vi "HFRR ADV v037 new software.vi"() -> ()   [LabVIEW 2025] (continued)
                      }
                      frame #18 {
                        n2411 = Wait (ms)(milliseconds to wait=u32 50) -> ()  [unwired: 1 out]
                      }
                      frame #19 {
                        n2412 = disable-structure shown="Disabled" {
                          frame Disabled {
                            n2413 = local read "EVENT LOG"() -> (w3480:string)
                            n2414 = call "Event Log.vi"("Content"="Test Parameter", "EVENT LOG"=w3480) -> ("EVENT LOG"=w3479:string)  [unwired: 8 in, 1 out]
                            n2415 = local write "EVENT LOG"(w3479) -> ()
                          }
                          frame Enabled {
                          }
                        }
                      }
                      frame #20 {
                        n2416 = Wait (ms)(milliseconds to wait=u32 50) -> ()  [unwired: 1 out]
                      }
                      frame #21 {
                        n2417 = local read "Set Hz"() -> (w3484:dbl)
                        n2418 = Number To Fractional String(number=w3484, precision (6)=i16 2) -> (F-format string=w3483:string)  [unwired: 2 in]
                        n2419 = Concatenate Strings("Set Frequency [Hz] :" ("Content"), w3483) -> (w3486:string)
                        n2420 = local read "EVENT LOG"() -> (w3488:string)
                        n2421 = call "Event Log.vi"("Content"=w3486, "EVENT LOG"=w3488) -> ("EVENT LOG"=w3487:string)  [unwired: 8 in, 1 out]
                        n2422 = local write "EVENT LOG"(w3487) -> ()
                      }
                      frame #22 {
                        n2423 = Wait (ms)(milliseconds to wait=u32 50) -> ()  [unwired: 1 out]
                      }
                      frame #23 {
                        n2424 = local read "NORMAL LOAD"() -> (w3491:dbl)
                        n2425 = Number To Fractional String(number=w3491, precision (6)=i16 2) -> (F-format string=w3492:string)  [unwired: 2 in]
                        n2426 = Concatenate Strings("Applied Load [grams] :" ("Content"), w3492) -> (w3494:string)
                        n2427 = local read "EVENT LOG"() -> (w3496:string)
                        n2428 = call "Event Log.vi"("Content"=w3494, "EVENT LOG"=w3496) -> ("EVENT LOG"=w3495:string)  [unwired: 8 in, 1 out]
                        n2429 = local write "EVENT LOG"(w3495) -> ()
                      }
                      frame #24 {
                        n2430 = Wait (ms)(milliseconds to wait=u32 50) -> ()  [unwired: 1 out]
                      }
                      frame #25 {
                        n2431 = local read "Set Strk"() -> (w3499:dbl)
                        n2432 = Number To Fractional String(number=w3499, precision (6)=i16 2) -> (F-format string=w3500:string)  [unwired: 2 in]
                        n2433 = Concatenate Strings("Set Stroke [mm] :" ("Content"), w3500) -> (w3502:string)
                        n2434 = local read "EVENT LOG"() -> (w3504:string)
                        n2435 = call "Event Log.vi"("Content"=w3502, "EVENT LOG"=w3504) -> ("EVENT LOG"=w3503:string)  [unwired: 8 in, 1 out]
                        n2436 = local write "EVENT LOG"(w3503) -> ()
                      }
                      frame #26 {
                        n2437 = Wait (ms)(milliseconds to wait=u32 50) -> ()  [unwired: 1 out]
                      }
                      frame #27 {
                        n2438 = local read "Set Temp"() -> (w3507:dbl)
                        n2439 = Number To Fractional String(number=w3507, precision (6)=i16 2) -> (F-format string=w3508:string)  [unwired: 2 in]
                        n2440 = Concatenate Strings("Set Temperature [deg C] :" ("Content"), w3508) -> (w3510:string)
                        n2441 = local read "EVENT LOG"() -> (w3512:string)
                        n2442 = call "Event Log.vi"("Content"=w3510, "EVENT LOG"=w3512) -> ("EVENT LOG"=w3511:string)  [unwired: 8 in, 1 out]
                        n2443 = local write "EVENT LOG"(w3511) -> ()
                      }
                      frame #28 {
                        n2444 = Wait (ms)(milliseconds to wait=u32 50) -> ()  [unwired: 1 out]
                      }
                      frame #29 {
                        n2445 = local read "Set Rh"() -> (w3515:dbl)
                        n2446 = Number To Fractional String(number=w3515, precision (6)=i16 2) -> (F-format string=w3516:string)  [unwired: 2 in]
                        n2447 = Concatenate Strings("Set Humidity [%RH] :" ("Content"), w3516) -> (w3518:string)
                        n2448 = local read "EVENT LOG"() -> (w3520:string)
                        n2449 = call "Event Log.vi"("Content"=w3518, "EVENT LOG"=w3520) -> ("EVENT LOG"=w3519:string)  [unwired: 8 in, 1 out]
                        n2450 = local write "EVENT LOG"(w3519) -> ()
                      }
                      frame #30 {
                        n2451 = Wait (ms)(milliseconds to wait=u32 50) -> ()  [unwired: 1 out]
                      }
                      frame #31 {
                        n2452 = local read "test time"() -> (w3523:dbl)
                        n2453 = Number To Fractional String(number=w3523, precision (6)=i16 1) -> (F-format string=w3524:string)  [unwired: 2 in]
                        n2454 = Concatenate Strings("Test Duration [mins] :" ("Content"), w3524) -> (w3526:string)
                        n2455 = local read "EVENT LOG"() -> (w3528:string)
                        n2456 = call "Event Log.vi"("Content"=w3526, "EVENT LOG"=w3528) -> ("EVENT LOG"=w3527:string)  [unwired: 8 in, 1 out]
                        n2457 = local write "EVENT LOG"(w3527) -> ()
                      }
                      frame #32 {
                        w3529 = dbl[] [] ("History Data")
                        w3530 = cluster{"y":dbl, dbl, "y":dbl}[] [] ("History Data")
                        w3531 = FALSE ("Visible")
                        n2458 = property on="Stroke ( mm )" class="WFChart (strict)"("History Data"=w3530) -> ()  [unwired: 2 in, 2 out]
                        n2459 = property on="Humidity ( %RH ) 2" class="WFChart (strict)"("History Data"=w3529) -> ()  [unwired: 2 in, 2 out]
                        n2460 = property on="Temperature ( Deg C )" class="WFChart (strict)"("History Data"=w3529) -> ()  [unwired: 2 in, 2 out]
                        n2461 = property on="Electrical Contact Resistance ( % )" class="WFChart (strict)"("History Data"=w3529) -> ()  [unwired: 2 in, 2 out]
                        n2462 = property on="Coefficient of Friction" class="WFChart (strict)"("History Data"=w3529) -> ()  [unwired: 2 in, 2 out]
                        n2463 = property on="Frictional Force ( N )" class="WFChart (strict)"("History Data"=w3529) -> ()  [unwired: 2 in, 2 out]
                        n2464 = property on="Coefficient of Friction" class="WFChart (strict)"("History Data"=w3529) -> ()  [unwired: 2 in, 2 out]
                        n2465 = property on="Frictional Force ( N )" class="WFChart (strict)"("History Data"=w3529) -> ()  [unwired: 2 in, 2 out]
                        n2466 = property on="Electrical Contact Resistance ( % )" class="WFChart (strict)"("History Data"=w3529) -> ()  [unwired: 2 in, 2 out]
                        n2467 = property on="Stroke ( mm )" class="WFChart (strict)"("History Data"=w3530) -> ()  [unwired: 2 in, 2 out]
                        n2468 = property on="Temperature ( Deg C )" class="WFChart (strict)"("History Data"=w3529) -> ()  [unwired: 2 in, 2 out]
                        n2469 = property on="Service Password Log" class="Str"("Visible"=w3531) -> ()  [unwired: 2 in, 2 out]
                        n2470 = property on="Password 3" class="Clust (strict)"("Visible"=w3531) -> ()  [unwired: 2 in, 2 out]
                      }
                    }
                    "TEST FILE NAM,E SAVED" <- TRUE ("TEST FILE NAM,E SAVED")
                  }
                }
              }
            }
          }
        }
        n2471 = local write "Test \nStatus"(w2910) -> ()
        n2472 = local write "Save"(w2910) -> ()
        n2473 = local read "Main Tab"() -> (w2904:T2)
        n2474 = case shown="True" w2907 {
          frame False {
            n2475 = local read "Rt 3"() -> (w2975:bool)
            n2476 = case shown="True" w2975 {
              frame False {
              }
              frame True {
                n2477 = local write "Rt 3"(FALSE ("Rt 3")) -> ()
              }
            }
            "Rt" <- TRUE ("Rt")
            "Rt 2" <- FALSE ("Rt")
          }
          frame True {
            n2478 = local read "Rt"() -> (w2981:bool)
            n2479 = local write "Rt 2"(TRUE ("Rt 2")) -> ()
            n2480 = case shown="True" w2981 {
              frame False {
              }
              frame True {
                n2481 = local write "Rt"(FALSE ("Rt")) -> ()
              }
            }
            "Rt 3" <- TRUE ("Rt 3")
          }
        }
        n2482 = case shown="\"Acquire\"" w2904 {
          tunnel: w2906 -> [_ w3010]
          frame Default {
            w3009 = 0.0 ("output")
            n2483 = local write "PID-out"(w3009) -> ()
            n2484 = local write "Frequency ( Hz )"(w3009) -> ()
            n2485 = local write "STROKE Initialize"(TRUE ("STROKE Initialize")) -> ()
          }
          frame "Acquire" {
            n2486 = stacked-sequence {
              frame #0 {
                n2487 = local read "Auto Start Test"() -> (w3012:bool)
                n2488 = case shown="True" w3012 {
                  tunnel: "RUN" -> [w3033 w3036]
                  tunnel: [w3033 w3035] -> w3013
                  frame False {
                  }
                  frame True {
                    n2489 = local read "Auto Start Temp"() -> (w3034:bool)
                    n2490 = Or(x=w3036, y=w3034) -> (x .or. y?=w3035:bool)
                  }
                }
                n2491 = local read "clk"() -> (w3032:dbl)
                n2492 = local read "Save"() -> (w3028:bool)
                n2493 = Equal?(x=w3032, y=0.0) -> (x = y?=w3029:bool)
                n2494 = And(x=w3029, y=w3028) -> (x .and. y?=w3030:bool)
                n2495 = Not(x="Engage") -> (.not. x?=w3019:bool)
                n2496 = case shown="False" w3013 {
                  tunnel: [0.0 w3059] -> w3015
                  frame False {
                    (unwired) TRUE ("Visible")
                    n2497 = local read "Auto Start Test"() -> (w3040:bool)
                    n2498 = local write "Start Time"(TRUE ("Start Time")) -> ()
                    n2499 = property on="Stroke 2" class="DigNum (strict)"("Visible"=FALSE) -> ()  [unwired: 2 in, 2 out]
                    n2500 = case shown="False" w3040 {
                      frame False {
                        n2501 = property on="Heater Button" class="Bool (strict)"("DisabledEnum"=T19."Enabled" ("Disabled")) -> ()  [unwired: 2 in, 2 out]
                        n2502 = property on="Humidity" class="Bool (strict)"("DisabledEnum"=T19."Enabled" ("Disabled")) -> ()  [unwired: 2 in, 2 out]
                      }
                      frame True {
                      }
                    }
                    n2503 = case shown="False" "TestCompFlg" {
                      frame False {
                        n2504 = local read "StartFlg"() -> (w3048:bool)
                        n2505 = case shown="True" w3048 {
                          frame False {
                          }
                          frame True {
                            n2506 = stacked-sequence {
                              frame #0 {
                                n2507 = local read "EVENT LOG"() -> (w3052:string)
                                n2508 = call "Event Log.vi"("Content"="Test was interrupted", "EVENT LOG"=w3052) -> ("EVENT LOG"=w3053:string)  [unwired: 8 in, 1 out]
                                n2509 = local write "EVENT LOG"(w3053) -> ()
                                n2510 = property on="RUN" class="Bool (strict)"("Visible"=TRUE) -> ()  [unwired: 2 in, 2 out]
                                n2511 = property on="Auto Start Test" class="Bool (strict)"("Visible"=TRUE) -> ()  [unwired: 2 in, 2 out]
                              }
                              frame #1 {
                                w3055 = FALSE ("StartFlg")
                                n2512 = property on="Heater Button" class="Bool (strict)"("Val(Sgnl)"=FALSE ("Value (Signaling)")) -> ()  [unwired: 2 in, 2 out]
                                n2513 = local write "Heater Button"(w3055) -> ()
                                n2514 = local write "StartFlg"(w3055) -> ()
                                n2515 = local write "Humidity"(w3055) -> ()
                              }
                              frame #2 {
                                n2516 = local write "Due Write"("VC;0" ("Command")) -> ()
                              }
                              frame #3 {
                                n2517 = Wait (ms)(milliseconds to wait=u32 1500) -> ()  [unwired: 1 out]
                              }
                              frame #4 {
                                n2518 = local write "Due Write"("HE;0" ("Command")) -> ()
                              }
                            }
                          }
                        }
                      }
                      frame True {
                      }
                    }
                    n2519 = local write "String 14"("Test will autostart once parameters reach the set value." ("String 14")) -> ()
                  }
                  frame True {
                    (unwired) FALSE ("Visible")
                    n2520 = property on="Stroke 2" class="DigNum (strict)"("Visible"=TRUE) -> ()  [unwired: 2 in, 2 out]
                    n2521 = property on="STOP 2" class="Bool (strict)"("Disabled"=u8 2) -> ()  [unwired: 2 in, 2 out]
                    n2522 = local write "String 14"(" Running....." ("String 14")) -> ()
                    n2523 = property on="Heater Button" class="Bool (strict)"("DisabledEnum"=T19."Disabled and Grayed Out" ("Disabled")) -> ()  [unwired: 2 in, 2 out]
                    n2524 = property on="Humidity" class="Bool (strict)"("DisabledEnum"=T19."Disabled and Grayed Out" ("Disabled")) -> ()  [unwired: 2 in, 2 out]
                    n2525 = case shown="True" "Start Time" {
                      selector: "Start Time" -> [_ w3078]
                      frame False {
                      }
                      frame True {
                        n2526 = Not(x=w3078) -> (.not. x?=w3077:bool)
                        n2527 = local write "Start Time"(w3077) -> ()
                        n2528 = local read "EVENT LOG"() -> (w3079:string)
                        n2529 = call "Event Log.vi"("Content"="Test in progress", "EVENT LOG"=w3079) -> ("EVENT LOG"=w3081:string)  [unwired: 8 in, 1 out]
                        n2530 = local write "EVENT LOG"(w3081) -> ()
                      }
                    }
                    n2531 = disable-structure shown="Enabled" {
                      disable-tunnel: [w3070 w3076] -> w3059
                      frame Disabled {
                        n2532 = local read "Set Hz"() -> (w3073:dbl)
                        n2533 = call <vilib>:"Uniform White Noise Waveform.vi"() -> ("signal out"=w3072:waveform(dbl))  [unwired: 10 in, 1 out]
                        n2534 = Random Number (0-1)() -> (number: 0 to 1=w3069:dbl)
                        n2535 = Add(x=w3073, y=w3072) -> (x+y=w3071:waveform(dbl))
                        n2536 = Multiply(x=ext 0.01 ("y"), y=w3069) -> (x*y=w3067:ext)
                        n2537 = Multiply(x=w3071, y=w3067) -> (x*y=w3070:waveform(ext))
                      }
                      frame Enabled {
                        n2538 = call-poly <vilib>:"Random Number (Range).vi"("lower bound (0)"=49.89, "upper bound (100)"=50.8) -> ("number"=w3076:dbl)  [unwired: 9 in]
                      }
                    }
                    "StartFlg" <- TRUE ("StartFlg")
                  }
                }
                n2539 = case shown="True" w3030 {
                  frame False {
                  }
                  frame True {
                    n2540 = local write "clk"(10.0 ("clk")) -> ()
                    n2541 = Get Date/Time In Seconds() -> (seconds since 1Jan1904=w3084:timestamp)
                    n2542 = To Double Precision Float(number=w3084) -> (double precision float=w3082:dbl)
                    n2543 = local write "acq timer"(w3082) -> ()
                    n2544 = local write "act save time"(w3082) -> ()
                  }
                }
                n2545 = call "Elapsed Time"("Time Target (s)"="Countdown", "Reset"=w3019) -> ("Elapsed Time (s)"=w3024:dbl, "Time has Elapsed"=w3022:bool)  [unwired: 10 in, 6 out]
                "Countdown 2" <- w3024
                n2546 = Subtract(x=w3024, y=2.0) -> (x-y=w3027:dbl)
                n2547 = Less?(x=w3027, y="Countdown") -> (x < y?=w3025:bool)
                n2548 = And(x=w3025, y=w3022) -> (x .and. y?=w3021:bool)
                n2549 = case shown="True" w3021 {
                  frame False {
                  }
                  frame True {
                    (unwired) dbl[] [] ("History Data")
                    n2550 = local write "Engage"(FALSE ("Engage")) -> ()
                    n2551 = local write "RUN"(TRUE ("RUN")) -> ()
                    n2552 = local read "Humidity ( %RH )"() -> (→"Rh Before":dbl)
                  }
                }
                n2553 = local read "Test \nStatus"() -> (w3017:bool)
                n2554 = Select(t=w3015, s=w3017, f=0.0) -> (s? t:f=w3016:dbl)
                n2555 = local write "Frequency ( Hz )"(w3016) -> ()
              }
              frame #1 {
                w3107 = 1000000.0 ("x")
                # "HC;1/0\nST;VALUE"
                # "Elapsed time\ncof\nstroke\nAir temp\nTemp\nHumidity"
                # "acq timer\n\nact save time"
                # "convert to microseconds"
                n2556 = local read "COUNT"() -> (w3090:i32)
                n2557 = local read "Rate"() -> (w3103:dbl)
                n2558 = Divide(x=w3107, y=w3103) -> (x/y=w3108:dbl)
                n2559 = Greater Or Equal?(x=w3090, y=250) -> (x >= y?=w3089:bool)
                n2560 = Get Date/Time In Seconds() -> (seconds since 1Jan1904=w3110:timestamp)
                n2561 = case shown="True" w3089 {
                  frame False {
                    n2562 = local read "COUNT"() -> (w3111:i32)
                    n2563 = Increment(x=w3111) -> (x+1=w3112:i32)
                    n2564 = local write "COUNT"(w3112) -> ()
                  }
                  frame True {
                    n2565 = local write "COUNT"(0 ("COUNT")) -> ()
                  }
                }
                n2566 = local read "Samplingtime 2"() -> (w3088:dbl)
                n2567 = local read "act save time"() -> (w3105:dbl)
                n2568 = Divide(x=w3108, y=w3107) -> (x/y=w3106:dbl)
                n2569 = To Double Precision Float(number=w3110) -> (double precision float=w3099:dbl)
                n2570 = Add(x=w3105, y=w3088) -> (x+y=w3104:dbl)
                n2571 = local read "acq timer"() -> (w3109:dbl)
                n2572 = local read "COUNT"() -> (w3092:i32)
                n2573 = Greater Or Equal?(x=w3099, y=w3104) -> (x >= y?=w3087:bool)
                n2574 = Multiply(x=w3106, y=w3092) -> (x*y=w3098:dbl)
                n2575 = Subtract(x=w3099, y=w3109) -> (x-y=w3101:dbl)
                n2576 = local read "Save"() -> (w3102:bool)
                n2577 = Add(x=w3101, y=w3098) -> (x+y=w3085:dbl)
                "Elapsed time 3" <- w3085
                n2578 = And(x=w3087, y=w3102) -> (x .and. y?=w3100:bool)
                n2579 = Divide(x=w3085, y=60.0) -> (x/y=w3096:dbl)
                n2580 = local read "Test \nStatus"() -> (w3086:bool)
                n2581 = local read "clk"() -> (w3093:dbl)
                n2582 = Equal?(x=w3093, y=10.0) -> (x = y?=w3095:bool)
                n2583 = case shown="True" w3100 {
                  tunnel: w3099 -> [_ w3231]
                  tunnel: [FALSE ("Boolean 2") TRUE ("Boolean 2")] -> _
                  frame False {
                  }
                  frame True {
                    w3185 = ";" ("Substring")
                    # "Pid out/\nFreq response value"
                    n2584 = local write "act save time"(w3231) -> ()
                    n2585 = local read "FILE"() -> (w3179:string)
                    n2586 = call "file check.vi"("file name in"=w3179) -> ("error out"=w3182:errorcluster, "file name out"=w3177:string)  [unwired: 9 in]
                    n2587 = local read "LVDT STROKE"() -> (w3174:dbl)
                    n2588 = local read "Add up Stroke"() -> (w3172:dbl)
                    n2589 = call "FILE PATH CREATION.vi"("error in"=w3182, "FILE NAME :"=w3177) -> ("FILE OUT"=w3180:path)  [unwired: 8 in, 1 out]
                    n2590 = local read "STROKE Initialize"() -> (w3167:bool)
                    n2591 = Concatenate Strings(w3177, ".dgf" ("Substring")) -> (w3181:string)
                    n2592 = Subtract(x=w3174, y=w3172) -> (x-y=w3173:dbl)
                    n2593 = Absolute Value(x=w3173) -> (abs(x)=w3170:dbl)
                    n2594 = local read "FF 2"() -> (→"Frictional Force ( N )" →"Frictional Force ( N )":dbl)
                    n2595 = Build Path(base path=w3180, name or relative path=w3181) -> (appended path=w3176:path)
                    n2596 = flat-sequence {
                      tunnel: w3170 -> [w3236]
                      tunnel: [w3235] -> w3168
                      tunnel: w3167 -> [w3233]
                      tunnel: [w3238] -> w3169
                      tunnel: w3168 -> [w3238]
                      frame #0 {
                        n2597 = call <vilib>:"Mean PtByPt.vi"("x"=w3236, "sample length"="STROKE FILTER", "initialize"=w3233) -> ("mean"=w3235:dbl)  [unwired: 1 in, 1 out]
                      }
                      frame #1 {
                        "STROKE Initialize" <- FALSE ("STROKE Initialize")
                      }
                    }
                    n2598 = local read "COF 2"() -> (w3190:dbl)
                    "Coefficient of Friction" <- w3190
                    "COF 4" <- w3190
                    "Coefficient of Friction" <- w3190
                    n2599 = local read "TEMP"() -> (w3193:dbl)
                    "Temperature ( Deg C )" <- w3193
                    n2600 = local read "Humidity ( %RH )"() -> (w3192:dbl)
                    "Humidity ( %RH ) 2" <- w3192
                    n2601 = local read "Frequency ( Hz )"() -> (w3199:dbl)
                    n2602 = local read "LVDT STROKE DISPLAY"() -> (w3171:dbl)
                    n2603 = local read "Elapsed time"() -> (w3224:dbl)
                    n2604 = local read "AIR TEMP"() -> (w3197:dbl)
                    n2605 = local read "PID-out"() -> (w3202:dbl)
                    n2606 = local write "Temperature ( Deg C )"(w3193) -> ()
                    n2607 = Number To Fractional String(number=w3171, width (-)=i16 9 ("precision (6)"), precision (6)=i16 6) -> (F-format string=w3217:string)  [unwired: 1 in]
                    n2608 = Number To Fractional String(number=w3197, width (-)=i16 9 ("precision (6)"), precision (6)=i16 3) -> (F-format string=w3216:string)  [unwired: 1 in]
                    n2609 = Number To Fractional String(number=w3193, width (-)=i16 9 ("precision (6)"), precision (6)=i16 3) -> (F-format string=w3213:string)  [unwired: 1 in]
                    n2610 = Number To Fractional String(number=w3192, width (-)=i16 9 ("precision (6)"), precision (6)=i16 3) -> (F-format string=w3210:string)  [unwired: 1 in]
                    n2611 = Number To Fractional String(number=0.0, width (-)=i16 9 ("precision (6)"), precision (6)=i16 3) -> (F-format string=w3207:string)  [unwired: 1 in]
                    n2612 = Number To Fractional String(number=w3202, width (-)=i16 9 ("precision (6)"), precision (6)=i16 3) -> (F-format string=w3203:string)  [unwired: 1 in]
                    n2613 = Number To Fractional String(number=w3199, width (-)=i16 9 ("precision (6)"), precision (6)=i16 3) -> (F-format string=w3198:string)  [unwired: 1 in]
                    n2614 = Number To Fractional String(number=w3190, width (-)=i16 9 ("precision (6)"), precision (6)=i16 6) -> (F-format string=w3225:string)  [unwired: 1 in]
                    n2615 = Number To Fractional String(number=w3224, width (-)=i16 14 ("precision (6)"), precision (6)=i16 3) -> (F-format string=w3226:string)  [unwired: 1 in]
                    n2616 = Bundle("y"=1.02, "LVDT STROKE DISPLAY"=w3171, "y"=0.98) -> (w3191:T30)  [unwired: 1 in]
                    n2617 = Number To Fractional String(number="Ambient Humidity :", width (-)=i16 9 ("precision (6)"), precision (6)=i16 6) -> (F-format string=w3183:string)  [unwired: 1 in]
                    n2618 = local read "RUN"() -> (w3189:bool)
                    n2619 = case shown="True" w3189 {
                      tunnel: w3191 -> [_ w3242]
                      tunnel: w3171 -> [_ w3241]
                      tunnel: w3171 -> [_ w3239]
                      tunnel: w3171 -> [_ w3240]
                      frame False {
                      }
                      frame True {
                        "Stroke ( mm )" <- w3242
                        "Stroke ( mm )" <- w3242
                        "Stroke 4" <- w3241
                        "Stroke 3" <- w3239
                        "Stroke 2" <- w3240
                        "measured_stroke" <- w3239
                      }
                    }
                    n2620 = Concatenate Strings(w3226, w3185, w3225, w3185, w3217, w3185, w3216, w3185, w3213, w3185, w3210, w3185, w3207, w3185, w3203, w3185, w3198, w3185, w3183, "\r") -> (w3223:string)
                    n2621 = call <vilib>:"Write Characters To File.vi"("append to file? (new file:F)"=TRUE, "character string"=w3223, "file path (dialog if empty)"=w3176) -> ()  [unwired: 2 in, 1 out]
                    "refresh flag" <- TRUE ("refresh flag")
                    "LVDT STROKE Actual" <- w3169
                  }
                }
                n2622 = case shown="True" w3086 {
                  tunnel: w3096 -> [_ w3122]
                  tunnel: w3101 -> [_ w3132]
                  tunnel: [0.0 w3128] -> _
                  tunnel: w3095 -> [_ w3127]
                  tunnel: [0.0 w3126] -> _
                  tunnel: w3085 -> [_ w3126]
                  tunnel: w3099 -> [w3115 _]
                  frame False {
                    n2623 = local write "acq timer"(w3115) -> ()
                    n2624 = local write "Test Duration Status"(0.0 ("Test Duration Status")) -> ()
                  }
                  frame True {
                    n2625 = local read "Set Hz"() -> (w3129:dbl)
                    n2626 = local write "Elapsed time"(w3122) -> ()
                    n2627 = local read "test time"() -> (w3121:dbl)
                    n2628 = Multiply(x=w3132, y=w3129) -> (x*y=w3131:dbl)
                    n2629 = case shown="False" w3127 {
                      tunnel: w3131 -> [w3133 _]
                      tunnel: [w3133 1.0] -> w3128
                      frame False {
                        n2630 = local write "Cycles elapsed"(w3133) -> ()
                      }
                      frame True {
                      }
                    }
                    n2631 = Greater?(x=w3122, y=w3121) -> (0:w3130:bool)
                    n2632 = Subtract(x=w3121, y=w3122) -> (x-y=w3120:dbl)
                    n2633 = Multiply(x=w3120, y=60.0) -> (x*y=w3119:dbl)
                    n2634 = local write "Time Remaining"(w3119) -> ()
                    n2635 = local write "Remaining Time"(w3119) -> ()
                    n2636 = case shown="True" w3130 {
                      frame False {
                      }
                      frame True {
                        n2637 = stacked-sequence {
                          frame #0 {
                            w3138 = T19."Enabled" ("Disabled")
                            w3137 = FALSE ("TEST FILE NAM,E SAVED")
                            w3139 = "" ("FILE")
                            w3140 = TRUE ("Visible")
                            n2638 = local write "Humidity"(FALSE ("Humidity")) -> ()
                            n2639 = local write "RUN"(FALSE ("OK Button 2")) -> ()
                            n2640 = local write "Heater Button"(FALSE ("Heater Button")) -> ()
                            n2641 = local write "Auto Start Test"(FALSE ("Auto Start Test")) -> ()
                            n2642 = local write "TestCompFlg"(TRUE ("StpFlg")) -> ()
                            n2643 = local read "Humidity ( %RH )"() -> (→"Rh After":dbl)
                            n2644 = property on="STOP 2" class="Bool (strict)"("Disabled"=u8 0) -> ()  [unwired: 2 in, 2 out]
                            n2645 = local read "EVENT LOG"() -> (w3145:string)
                            n2646 = call "Event Log.vi"("Content"="Test Completed", "EVENT LOG"=w3145) -> ("EVENT LOG"=w3144:string)  [unwired: 8 in, 1 out]
                            n2647 = property on="RUN" class="Bool (strict)"("Visible"=w3140) -> ()  [unwired: 2 in, 2 out]
                            n2648 = property on="Auto Start Test" class="Bool (strict)"("Visible"=w3140) -> ()  [unwired: 2 in, 2 out]
                            n2649 = local write "Batch Ref Num :"(w3139) -> ()
                            n2650 = local write "FILE"(w3139) -> ()
                            n2651 = local write "EVENT LOG"(w3144) -> ()
                            n2652 = local write "TEST FILE NAM,E SAVED"(w3137) -> ()
                            n2653 = local write "Fuel Discription :"(w3139) -> ()
                            n2654 = local write "START TEMP"(w3137) -> ()
                            n2655 = local write "Remarks :"(w3139) -> ()
                            n2656 = local write "Main Dashboard Buttons"(T1."Imaging" ("Main Dashboard Buttons")) -> ()
                            n2657 = local write "Main Tab"(T2."Adv Scar" ("Main Tab")) -> ()
                            n2658 = property on="FRICVALZ 2" class="Bool (strict)"("DisabledEnum"=w3138) -> ()  [unwired: 2 in, 2 out]
                            n2659 = property on="FRICVALZ 3" class="Bool (strict)"("DisabledEnum"=w3138) -> ()  [unwired: 2 in, 2 out]
                            n2660 = property on="FRICVALZ 4" class="Bool (strict)"("DisabledEnum"=w3138) -> ()  [unwired: 2 in, 2 out]
                          }
                          frame #1 {
                            n2661 = Wait (ms)(milliseconds to wait=u32 1500) -> ()  [unwired: 1 out]
                          }
                          frame #2 {
                            n2662 = local read "WriteHumidity"() -> (w3154:string[])
                            n2663 = Insert Into Array(array=w3154, new element="R;1" ("new element/subarray")) -> (w3152:string[])  [unwired: 1 in]
                            n2664 = local write "Due Write"("VC;0") -> ()
                            n2665 = local write "WriteHumidity"(w3152) -> ()
                          }
                          frame #3 {
                            n2666 = Wait (ms)(milliseconds to wait=u32 1500) -> ()  [unwired: 1 out]
                          }
                          frame #4 {
                            n2667 = local read "WriteHumidity"() -> (w3159:string[])
                            n2668 = Insert Into Array(array=w3159, new element="R;1" ("new element/subarray")) -> (w3158:string[])  [unwired: 1 in]
                            n2669 = local write "Due Write"("VC;0") -> ()
                            n2670 = local write "WriteHumidity"(w3158) -> ()
                          }
                          frame #5 {
                            n2671 = Wait (ms)(milliseconds to wait=u32 1500) -> ()  [unwired: 1 out]
                          }
                          frame #6 {
                            n2672 = local write "Due Write"("ST;0") -> ()
                          }
                          frame #7 {
                            n2673 = local write "measured_stroke"(0.0 ("measured_stroke")) -> ()
                            n2674 = Wait (ms)(milliseconds to wait=u32 1500) -> ()  [unwired: 1 out]
                          }
                          frame #8 {
                            n2675 = local write "Due Write"("HE;0") -> ()
                          }
                        }
                      }
                    }
                    n2676 = Divide(x=w3122, y=w3121) -> (x/y=w3125:dbl)
                    n2677 = Multiply(x=w3125, y=100.0) -> (x*y=w3123:dbl)
                    n2678 = local write "Test Duration Status"(w3123) -> ()
                  }
                }
              }
              frame #2 {
                n2679 = case shown="True" "Heater Button" {
                  tunnel: [0.0 ("output") w3265] -> w3243
                  frame False {
                    w3246 = TRUE ("tmpchk")
                    n2680 = local read "TEMP"() -> (w3247:dbl)
                    n2681 = local write "Temp ini"(w3247) -> ()
                    n2682 = local write "Reset 4"(w3246) -> ()
                    n2683 = local write "tmpchk"(w3246) -> ()
                    n2684 = local write "reinit"(TRUE ("reinit")) -> ()
                    n2685 = local write "manual temp log"(TRUE ("manual temp log")) -> ()
                  }
                  frame True {
                    # "Logic to turn off\nthe heater when \ntemp is not rising.\nTime - 60 sec\nDelta t- 5°c"
                    n2686 = local read "Temp ini"() -> (w3254:dbl)
                    n2687 = local read "Auto Start Test"() -> (w3250:bool)
                    n2688 = Less?(x=w3254, y=53.0) -> (x < y?=w3252:bool)
                    n2689 = case shown="False" w3250 {
                      frame False {
                        n2690 = local read "Set Temp"() -> (w3274:dbl)
                        n2691 = local read "TEMP"() -> (w3273:dbl)
                        n2692 = Subtract(x=w3274, y=w3273) -> (x-y=w3272:dbl)
                        n2693 = Absolute Value(x=w3272) -> (abs(x)=w3271:dbl)
                        n2694 = Less?(x=w3271, y=0.5) -> (x < y?=w3269:bool)
                        n2695 = case shown="True" w3269 {
                          tunnel: "manual temp log" -> [_ w3275]
                          frame False {
                          }
                          frame True {
                            n2696 = case shown="True" w3275 {
                              selector: w3275 -> [_ w3276]
                              frame False {
                              }
                              frame True {
                                # "#Event log"
                                n2697 = Not(x=w3276) -> (.not. x?=w3277:bool)
                                n2698 = local write "manual temp log"(w3277) -> ()
                                n2699 = local read "EVENT LOG"() -> (w3280:string)
                                n2700 = call "Event Log.vi"("Content"="Target Temperature reached", "EVENT LOG"=w3280) -> ("EVENT LOG"=w3279:string)  [unwired: 8 in, 1 out]
                                n2701 = local write "EVENT LOG"(w3279) -> ()
                              }
                            }
                          }
                        }
                      }
                      frame True {
                        n2702 = local write "manual temp log"(TRUE ("manual temp log")) -> ()
                      }
                    }
                    n2703 = And(x="tmpchk", y=w3252) -> (x .and. y?=w3255:bool)
                    n2704 = case shown="True" w3255 {
                      frame False {
                      }
                      frame True {
                        n2705 = call "Elapsed Time8"("Time Target (s)"=300.0, "Reset"="Reset 4") -> ("Time has Elapsed"=w3282:bool)  [unwired: 10 in, 7 out]
                        n2706 = flat-sequence {
                          tunnel: w3282 -> [_]
                          frame #0 {
                            n2707 = local write "Reset 4"(FALSE ("Reset 4")) -> ()
                          }
                        }
                        n2708 = case shown="True" w3282 {
                          frame False {
                          }
                          frame True {
                            n2709 = local read "Temp ini"() -> (w3289:dbl)
                            n2710 = Add(x=w3289, y=5.0) -> (x+y=w3287:dbl)
                            n2711 = local read "TEMP"() -> (w3290:dbl)
                            n2712 = Greater?(x=w3290, y=w3287) -> (0:w3288:bool)
                            n2713 = case shown="False" w3288 {
                              frame False {
                                n2714 = local write "Heater Button"(FALSE ("Heater Button")) -> ()
                              }
                              frame True {
                                n2715 = local write "tmpchk"(FALSE ("tmpchk")) -> ()
                              }
                            }
                          }
                        }
                      }
                    }
                    n2716 = local read "Set Temp"() -> (w3263:dbl)
                    n2717 = local read "TEMP"() -> (w3257:dbl)
                    n2718 = call-poly <vilib>:"PID.vi"("reinitialize? (F)"="reinit", "dt (s)"=-1.0, "process variable"=w3257, "setpoint"=w3263) -> ("output"=w3260:dbl)  [unwired: 6 in, 1 out]
                    n2719 = Subtract(x=w3263, y=w3257) -> (x-y=w3264:dbl)
                    n2720 = Add(x=w3263, y=0.5) -> (x+y=w3261:dbl)
                    n2721 = Greater Or Equal?(x=w3257, y=w3261) -> ()  [unwired: 1 out]
                    n2722 = Select(t=0.0, s=FALSE, f=w3260) -> (s? t:f=w3259:dbl)
                    "PID output" <- w3259
                    n2723 = flat-sequence {
                      tunnel: w3259 -> [w3293]
                      tunnel: [w3293] -> w3265
                      frame #0 {
                        n2724 = local write "reinit"(FALSE ("reinit")) -> ()
                      }
                    }
                    n2725 = Bundle(w3264, "output"=w3259, "TEMP"=w3257) -> ()  [unwired: 1 in, 1 out]
                  }
                }
                "PID-out" <- w3243
              }
              frame #3 {
                n2726 = local read "TEMP"() -> (w3295:dbl)
                n2727 = Greater Or Equal?(x=w3295, y="Set Temp 2") -> (x >= y?=w3300:bool)
                n2728 = case shown="True" w3300 {
                  tunnel: [FALSE TRUE] -> w3298
                  frame False {
                  }
                  frame True {
                  }
                }
                "Status 13" <- w3298
                n2729 = And(x=w3298, y="trip1 8") -> (x .and. y?=w3297:bool)
                n2730 = case shown="True" w3297 {
                  frame False {
                    n2731 = local write "Heater Trip Temp"(TRUE ("Heater Trip Temp")) -> ()
                  }
                  frame True {
                    w3303 = FALSE ("OK Button 2")
                    n2732 = case shown="True" "Heater Trip Temp" {
                      selector: "Heater Trip Temp" -> [_ w3305]
                      frame False {
                      }
                      frame True {
                        n2733 = Not(x=w3305) -> (.not. x?=w3304:bool)
                        n2734 = local read "EVENT LOG"() -> (w3308:string)
                        n2735 = local write "Heater Trip Temp"(w3304) -> ()
                        n2736 = call "Event Log.vi"("Content"="Heater Trip", "EVENT LOG"=w3308) -> ("EVENT LOG"=w3307:string)  [unwired: 8 in, 1 out]
                        n2737 = local write "EVENT LOG"(w3307) -> ()
                      }
                    }
                    n2738 = local write "RUN"(w3303) -> ()
                    n2739 = property on="Auto Start Test" class="Bool (strict)"("Value"=w3303) -> ()  [unwired: 2 in, 2 out]
                    n2740 = local write "Heater Button"(w3303) -> ()
                  }
                }
              }
            }
            n2741 = case shown="False" w3010 {
              frame False {
                n2742 = disable-structure shown="Disabled" {
                  frame Disabled {
                    n2743 = stacked-sequence {
                      frame #0 {
                        n2744 = local write "RUN"(FALSE ("OK Button 2")) -> ()
                      }
                      frame #1 {
                      }
                    }
                  }
                  frame Enabled {
                  }
                }
              }
              frame True {
              }
            }
          }
        }
        n2745 = local read "Reset Graph"() -> (w2903:bool)
        n2746 = case shown="True" w2903 {
          selector: w2903 -> [_ w2920]
          frame False {
          }
          frame True {
            w2934 = 0.0 ("X Scale.Range:Maximum")
            n2747 = Not(x=w2920) -> (.not. x?=w2919:bool)
            n2748 = local write "Reset Graph"(w2919) -> ()
            n2749 = property on="Electrical Contact Resistance ( % )" class="WFChart (strict)"("XScale.Maximum"=600.0 ("X Scale.Range:Maximum"), "XScale.Minimum"=0.0 ("X Scale.Range:Minimum"), "YScale.Maximum"=100.0 ("Y Scale.Range:Maximum"), "YScale.Minimum"=0.0 ("Y Scale.Range:Minimum")) -> ()  [unwired: 2 in, 2 out]
            n2750 = property on="Frictional Force ( N )" class="WFChart (strict)"("XScale.Maximum"=600.0 ("X Scale.Range:Maximum"), "XScale.Minimum"=0.0 ("X Scale.Range:Minimum"), "YScale.Maximum"=100.0 ("Y Scale.Range:Maximum"), "YScale.Minimum"=0.0 ("Y Scale.Range:Minimum")) -> ()  [unwired: 2 in, 2 out]
            n2751 = property on="Temperature ( Deg C )" class="WFChart (strict)"("XScale.Maximum"=600.0 ("X Scale.Range:Maximum"), "XScale.Minimum"=0.0 ("X Scale.Range:Minimum"), "YScale.Maximum"=100.0 ("Y Scale.Range:Maximum"), "YScale.Minimum"=0.0 ("Y Scale.Range:Minimum")) -> ()  [unwired: 2 in, 2 out]
            n2752 = property on="Stroke ( mm )" class="WFChart (strict)"("XScale.Maximum"=600.0 ("X Scale.Range:Maximum"), "XScale.Minimum"=0.0 ("X Scale.Range:Minimum"), "YScale.Maximum"=100.0 ("Y Scale.Range:Maximum"), "YScale.Minimum"=0.0 ("Y Scale.Range:Minimum")) -> ()  [unwired: 2 in, 2 out]
            n2753 = property on="Coefficient of Friction" class="WFChart (strict)"("XScale.Maximum"=600.0 ("X Scale.Range:Maximum"), "XScale.Minimum"=0.0 ("X Scale.Range:Minimum"), "YScale.Maximum"=100.0 ("Y Scale.Range:Maximum"), "YScale.Minimum"=0.0 ("Y Scale.Range:Minimum")) -> ()  [unwired: 2 in, 2 out]
            n2754 = property on="Electrical Contact Resistance ( % )" class="WFChart (strict)"("XScale.Minimum"=0.0 ("X Scale.Range:Minimum"), "XScale.Maximum"=600.0 ("X Scale.Range:Maximum"), "YScale.Minimum"=0.0 ("Y Scale.Range:Minimum"), "YScale.Maximum"=100.0 ("Y Scale.Range:Maximum")) -> ()  [unwired: 2 in, 2 out]
            n2755 = property on="Temperature ( Deg C )" class="WFChart (strict)"("XScale.Minimum"=0.0 ("X Scale.Range:Minimum"), "XScale.Maximum"=600.0 ("X Scale.Range:Maximum"), "YScale.Minimum"=0.0 ("Y Scale.Range:Minimum"), "YScale.Maximum"=100.0 ("Y Scale.Range:Maximum")) -> ()  [unwired: 2 in, 2 out]
            n2756 = property on="Coefficient of Friction" class="WFChart (strict)"("XScale.Minimum"=0.0 ("X Scale.Range:Minimum"), "XScale.Maximum"=600.0 ("X Scale.Range:Maximum"), "YScale.Maximum"=1.0 ("X Scale.Range:Minimum"), "YScale.Minimum"=0.0 ("X Scale.Range:Minimum")) -> ()  [unwired: 2 in, 2 out]
            n2757 = property on="Frictional Force ( N )" class="WFChart (strict)"("XScale.Maximum"=600.0 ("X Scale.Range:Maximum"), "XScale.Minimum"=w2934, "YScale.Maximum"=10.0 ("Y Scale.Range:Maximum"), "YScale.Minimum"=w2934) -> ()  [unwired: 2 in, 2 out]
            n2758 = property on="Stroke ( mm )" class="WFChart (strict)"("XScale.Maximum"=600.0 ("X Scale.Range:Maximum"), "XScale.Minimum"=0.0 ("X Scale.Range:Minimum"), "YScale.Maximum"=100.0 ("Y Scale.Range:Maximum"), "YScale.Minimum"=0.0 ("Y Scale.Range:Minimum")) -> ()  [unwired: 2 in, 2 out]
            n2759 = property on="Humidity ( %RH ) 2" class="WFChart (strict)"("XScale.Maximum"=600.0 ("X Scale.Range:Maximum"), "XScale.Minimum"=0.0 ("X Scale.Range:Minimum"), "YScale.Maximum"=100.0 ("Y Scale.Range:Maximum"), "YScale.Minimum"=0.0 ("Y Scale.Range:Minimum")) -> ()  [unwired: 2 in, 2 out]
          }
        }
      }
      frame "Compare Files" {
        # "Elapsed time\ncof\nstroke\nAir temp\nTemp\nHumidity"
        n2760 = case shown="True" "RSTV1 2" {
          frame False {
          }
          frame True {
            n2761 = property on="Humidity ( %RH )" class="XYGraph (strict)"("Y Scale.Display Format:Precision"=u8 0 ("Y Scale.Format & Precision:Precision")) -> ()  [unwired: 2 in, 2 out]
            n2762 = property on="Humidity ( %RH )" class="XYGraph (strict)"("X Scale.Range:Minimum"=0.0, "X Scale.Range:Maximum"=75.0, "Y Scale.Range:Minimum"=48.0, "Y Scale.Range:Maximum"=58.0) -> ()  [unwired: 2 in, 2 out]
          }
        }
        n2763 = case shown="True" "RST CP 2" {
          frame False {
          }
          frame True {
            n2764 = property on="XY Graph 13" class="XYGraph (strict)"("Y Scale.Display Format:Precision"=u8 0 ("Y Scale.Format & Precision:Precision")) -> ()  [unwired: 2 in, 2 out]
            n2765 = property on="XY Graph 13" class="XYGraph (strict)"("X Scale.Range:Minimum"=0.0, "X Scale.Range:Maximum"=75.0, "Y Scale.Range:Minimum"=0.0, "Y Scale.Range:Maximum"=100.0) -> ()  [unwired: 2 in, 2 out]
          }
        }
        n2766 = case shown="True" "RST CP" {
          frame False {
          }
          frame True {
            n2767 = property on="Sample Temperature ( °C )" class="XYGraph (strict)"("Y Scale.Display Format:Precision"=u8 2 ("Y Scale.Format & Precision:Precision")) -> ()  [unwired: 2 in, 2 out]
            n2768 = property on="Sample Temperature ( °C )" class="XYGraph (strict)"("X Scale.Range:Minimum"=0.0, "X Scale.Range:Maximum"=75.0, "Y Scale.Range:Minimum"=58.0, "Y Scale.Range:Maximum"=62.0) -> ()  [unwired: 2 in, 2 out]
          }
        }
        n2769 = case shown="True" "RSTV1 3" {
          frame False {
          }
          frame True {
            n2770 = property on="Air Temperature  ( °C )" class="XYGraph (strict)"("Y Scale.Display Format:Precision"=u8 2 ("Y Scale.Format & Precision:Precision")) -> ()  [unwired: 2 in, 2 out]
            n2771 = property on="Air Temperature  ( °C )" class="XYGraph (strict)"("X Scale.Range:Minimum"=0.0 ("Y Scale.Range:Minimum"), "X Scale.Range:Maximum"=75.0 ("Y Scale.Range:Maximum"), "Y Scale.Range:Minimum"=20.0 ("X Scale.Range:Minimum"), "Y Scale.Range:Maximum"=26.0 ("X Scale.Range:Maximum")) -> ()  [unwired: 2 in, 2 out]
          }
        }
        n2772 = case shown="True" "RSTV1 4" {
          frame False {
          }
          frame True {
            n2773 = property on="Stroke ( mm )" class="XYGraph (strict)"("Y Scale.Display Format:Precision"=u8 2 ("Y Scale.Format & Precision:Precision")) -> ()  [unwired: 2 in, 2 out]
            n2774 = property on="Stroke ( mm )" class="XYGraph (strict)"("X Scale.Range:Minimum"=0.0 ("Y Scale.Range:Maximum"), "X Scale.Range:Maximum"=75.0 ("X Scale.Range:Minimum"), "Y Scale.Range:Minimum"=0.98, "Y Scale.Range:Maximum"=1.02) -> ()  [unwired: 2 in, 2 out]
          }
        }
        n2775 = case shown="True" "rstv2" {
          frame False {
          }
          frame True {
            n2776 = property on="Coefficient Of Friction" class="XYGraph (strict)"("Y Scale.Display Format:Precision"=u8 3 ("Y Scale.Format & Precision:Precision")) -> ()  [unwired: 2 in, 2 out]
            n2777 = property on="Coefficient Of Friction" class="XYGraph (strict)"("X Scale.Range:Minimum"=0.0 ("Y Scale.Range:Maximum"), "X Scale.Range:Maximum"=75.0, "Y Scale.Range:Minimum"=0.0, "Y Scale.Range:Maximum"=1.0 ("X Scale.Range:Minimum")) -> ()  [unwired: 2 in, 2 out]
          }
        }
        n2778 = case shown="True" "RST CP 3" {
          frame False {
          }
          frame True {
            n2779 = property on="Air Temp ( °C ) vs Humidity ( % RH )" class="XYGraph (strict)"("X Scale.Range:Minimum"=18.0, "X Scale.Range:Maximum"=28.0 ("X Scale.Range:Minimum"), "Y Scale.Range:Minimum"=30.0 ("X Scale.Range:Minimum"), "Y Scale.Range:Maximum"=70.0 ("X Scale.Range:Minimum")) -> ()  [unwired: 2 in, 2 out]
          }
        }
        n2780 = case shown="True" "OPEN 1" {
          frame False {
          }
          frame True {
            (unwired) 0  # existing file
            w3584 = "Choose a datalog file to open"  # prompt
            n2781 = local write "OPEN 1"(FALSE ("OPEN 1")) -> ()
            n2782 = String To Path(string="C:\\LAB-IQ\\Data\\") -> (path=w3569:path)
            n2783 = File Dialog(6:"*.dgf" ("pattern"), 7:w3584, 11:w3569) -> (0:w3567:errorcluster, 3:w3575:path)  [unwired: 4 in, 2 out]
            n2784 = Unbundle(w3567) -> ()  [unwired: 3 out]
            n2785 = Strip Path(path=w3575) -> (name=w3574:string)  [unwired: 1 out]
            n2786 = Path To String(path=w3575) -> (string=w3570:string)
            "string1" <- w3570
            n2787 = Match Pattern(string=w3574, regular expression=".dgf") -> (before substring=→"String Control":string)  [unwired: 1 in, 3 out]
            n2788 = Match Pattern(string=w3570, regular expression=".dgf" ("substring (\"\")")) -> (before substring=w3580:string)  [unwired: 1 in, 3 out]
            n2789 = Concatenate Strings(w3580, ".duf" ("Substring")) -> (w3576:string)
            n2790 = String To Path(string=w3576) -> (path=w3581:path)
            n2791 = call <vilib>:"Read Characters From File.vi"("file path (dialog if empty)"=w3581, "start of read offset (chars.:0)"=60 ("start of read offset (chars.: 0)")) -> ("character string"=→"String Control 2":string)  [unwired: 4 in, 3 out]
          }
        }
        n2792 = case shown="True" "OPEN 2" {
          frame False {
          }
          frame True {
            (unwired) 0  # existing file
            w3602 = "Choose a datalog file to open"  # prompt
            n2793 = local write "OPEN 2"(FALSE ("OPEN 1")) -> ()
            n2794 = String To Path(string="C:\\LAB-IQ\\Data\\") -> (path=w3587:path)
            n2795 = File Dialog(6:"*.dgf" ("pattern"), 7:w3602, 11:w3587) -> (0:w3585:errorcluster, 3:w3593:path)  [unwired: 4 in, 2 out]
            n2796 = Unbundle(w3585) -> ()  [unwired: 3 out]
            n2797 = Strip Path(path=w3593) -> (name=w3591:string)  [unwired: 1 out]
            n2798 = Path To String(path=w3593) -> (string=w3588:string)
            "string1 2" <- w3588
            n2799 = Match Pattern(string=w3591, regular expression=".dgf") -> (before substring=→"String Control 3":string)  [unwired: 1 in, 3 out]
            n2800 = Match Pattern(string=w3588, regular expression=".dgf" ("substring (\"\")")) -> (before substring=w3599:string)  [unwired: 1 in, 3 out]
            n2801 = Concatenate Strings(w3599, ".duf" ("Substring")) -> (w3596:string)
            n2802 = String To Path(string=w3596) -> (path=w3594:path)
            n2803 = call <vilib>:"Read Characters From File.vi"("file path (dialog if empty)"=w3594, "start of read offset (chars.:0)"=60 ("start of read offset (chars.: 0)")) -> ("character string"=→"String Control 4":string)  [unwired: 4 in, 3 out]
          }
        }
        n2804 = case shown="True" "OPEN 3" {
          frame False {
          }
          frame True {
            (unwired) 0  # existing file
            w3620 = "Choose a datalog file to open"  # prompt
            n2805 = local write "OPEN 3"(FALSE ("OPEN 1")) -> ()
            n2806 = String To Path(string="C:\\LAB-IQ\\Data\\") -> (path=w3605:path)
            n2807 = File Dialog(6:"*.dgf" ("pattern"), 7:w3620, 11:w3605) -> (0:w3603:errorcluster, 3:w3611:path)  [unwired: 4 in, 2 out]
            n2808 = Unbundle(w3603) -> ()  [unwired: 3 out]
            n2809 = Strip Path(path=w3611) -> (name=w3609:string)  [unwired: 1 out]
            n2810 = Path To String(path=w3611) -> (string=w3606:string)
            "string1 3" <- w3606
            n2811 = Match Pattern(string=w3609, regular expression=".dgf") -> (before substring=→"String Control 5":string)  [unwired: 1 in, 3 out]
            n2812 = Match Pattern(string=w3606, regular expression=".dgf" ("substring (\"\")")) -> (before substring=w3616:string)  [unwired: 1 in, 3 out]
            n2813 = Concatenate Strings(w3616, ".duf" ("Substring")) -> (w3613:string)
            n2814 = String To Path(string=w3613) -> (path=w3617:path)
            n2815 = call <vilib>:"Read Characters From File.vi"("file path (dialog if empty)"=w3617, "start of read offset (chars.:0)"=60 ("start of read offset (chars.: 0)")) -> ("character string"=→"String Control 6":string)  [unwired: 4 in, 3 out]
          }
        }
        n2816 = case shown="True" "OPEN 4" {
          frame False {
          }
          frame True {
            (unwired) 0  # existing file
            w3638 = "Choose a datalog file to open"  # prompt
            n2817 = local write "OPEN 4"(FALSE ("OPEN 1")) -> ()
            n2818 = String To Path(string="C:\\LAB-IQ\\Data\\") -> (path=w3623:path)
            n2819 = File Dialog(6:"*.dgf" ("pattern"), 7:w3638, 11:w3623) -> (0:w3621:errorcluster, 3:w3629:path)  [unwired: 4 in, 2 out]
            n2820 = Unbundle(w3621) -> ()  [unwired: 3 out]
            n2821 = Strip Path(path=w3629) -> (name=w3627:string)  [unwired: 1 out]
            n2822 = Path To String(path=w3629) -> (string=w3624:string)
            "string1 4" <- w3624
            n2823 = Match Pattern(string=w3627, regular expression=".dgf") -> (before substring=→"String Control 7":string)  [unwired: 1 in, 3 out]
            n2824 = Match Pattern(string=w3624, regular expression=".dgf" ("substring (\"\")")) -> (before substring=w3634:string)  [unwired: 1 in, 3 out]
            n2825 = Concatenate Strings(w3634, ".duf" ("Substring")) -> (w3631:string)
            n2826 = String To Path(string=w3631) -> (path=w3635:path)
            n2827 = call <vilib>:"Read Characters From File.vi"("file path (dialog if empty)"=w3635, "start of read offset (chars.:0)"=60 ("start of read offset (chars.: 0)")) -> ("character string"=→"String Control 8":string)  [unwired: 4 in, 3 out]
          }
        }
      }
      frame "About" {
        # "Elapsed time\ncof\nstroke\nmean pos\nTemp\nHumidity"
        n2828 = disable-structure shown="Disabled" {
          frame Disabled {
            n2829 = case shown="True" "Export" {
              frame False {
              }
              frame True {
                w3660 = "                                      " ("string")
                w3662 = "\r"
                (unwired) i16 6 ("width (-)")
                w3739 = "\r"
                w3671 = "\r"
                n2830 = local write "Export"(FALSE ("Export")) -> ()
                n2831 = local read "String 29"() -> (w3708:string)
                n2832 = local read "String 34"() -> (w3696:string)
                n2833 = local read "String 35"() -> (w3691:string)
                n2834 = local read "String 37"() -> (w3687:string)
                n2835 = local read "String 36"() -> (w3684:string)
                n2836 = local read "String 38"() -> (w3681:string)
                n2837 = local read "String 39"() -> (w3678:string)
                n2838 = Match Pattern(string=w3708, regular expression=".dwm") -> (before substring=w3704:string)  [unwired: 1 in, 3 out]
                "before substring" <- w3704
                n2839 = local read "S 38"() -> (w3699:string)
                n2840 = local read "S 39"() -> (w3692:string)
                n2841 = local read "Temperature before test 2"() -> (w3728:dbl)
                n2842 = local read "Temperature after test 2"() -> (w3733:dbl)
                n2843 = local read "Humidity before test 2"() -> (w3714:dbl)
                n2844 = local read "Humidity after test 2"() -> (w3729:dbl)
                n2845 = local read "MWSD 2"() -> (w3725:dbl)
                n2846 = local read "WS1.4 2"() -> (w3741:dbl)
                n2847 = local read "HCF 2"() -> (w3737:dbl)
                n2848 = local read "AVP 2"() -> (w3726:dbl)
                n2849 = Concatenate Strings("1," ("string"), w3699) -> (w3698:string)
                n2850 = Concatenate Strings("2," ("string"), w3696) -> (w3695:string)
                n2851 = Concatenate Strings("3," ("string"), w3692) -> (w3694:string)
                n2852 = Concatenate Strings("4," ("string"), w3691) -> (w3690:string)
                n2853 = Concatenate Strings("5," ("string"), w3687) -> (w3688:string)
                n2854 = Concatenate Strings("6," ("string"), w3684) -> (w3685:string)
                n2855 = Concatenate Strings("7," ("string"), w3681) -> (w3682:string)
                n2856 = Concatenate Strings("8," ("string"), w3678) -> (w3679:string)
                n2857 = local read "Sample ID"() -> (w3746:string)
                n2858 = case shown="\"xlx\"" "Select File Type" {
                  tunnel: w3704 -> [w3749 w3751 w3753]
                  tunnel: [w3747 w3752 w3754] -> w3703
                  frame "xlx" {
                    n2859 = Concatenate Strings(w3749, ".xls" ("string")) -> (w3747:string)
                  }
                  frame "csv" {
                    n2860 = Concatenate Strings(w3751, ".csv" ("string")) -> (w3752:string)
                  }
                  frame "txt" {
                    n2861 = Concatenate Strings(w3753, ".txt" ("string")) -> (w3754:string)
                  }
                }
                n2862 = local read "Test Date"() -> (w3745:string)
                n2863 = local read "String 45"() -> (w3659:string)
                n2864 = local read "String 31"() -> (w3744:string)
                n2865 = local read "String 32"() -> (w3743:string)
                n2866 = local read "TITTLE"() -> (w3667:string)
                n2867 = Number To Fractional String(number=w3714, width (-)=i16 6, precision (6)=i16 2) -> (F-format string=w3713:string)  [unwired: 1 in]
                n2868 = Number To Fractional String(number=w3728, width (-)=i16 6, precision (6)=i16 2) -> (F-format string=w3734:string)  [unwired: 1 in]
                n2869 = Number To Fractional String(number=w3729, width (-)=i16 6, precision (6)=i16 2) -> (F-format string=w3727:string)  [unwired: 1 in]
                n2870 = Number To Fractional String(number=w3733, width (-)=i16 6, precision (6)=i16 2) -> (F-format string=w3732:string)  [unwired: 1 in]
                n2871 = Number To Fractional String(number=w3725, width (-)=i16 6, precision (6)=i16 2) -> (F-format string=w3723:string)  [unwired: 1 in]
                n2872 = Number To Fractional String(number=w3726, width (-)=i16 6, precision (6)=i16 2) -> (F-format string=w3724:string)  [unwired: 1 in]
                n2873 = Number To Fractional String(number=w3737, width (-)=i16 6, precision (6)=i16 2) -> (F-format string=w3738:string)  [unwired: 1 in]
                n2874 = Number To Fractional String(number=w3741, precision (6)=i16 2) -> (F-format string=w3742:string)  [unwired: 2 in]
                n2875 = local read "s.NO"() -> (w3661:string)
                n2876 = Concatenate Strings("=" ("string"), w3667) -> (w3666:string)
                n2877 = Concatenate Strings("S.No," ("string"), "                                       Parameters" ("string")) -> (w3672:string)
                n2878 = Concatenate Strings(w3739, w3698, w3713, w3739, w3695, w3734, w3739, w3694, w3727, w3739, w3690, w3732, w3739, w3688, w3723, w3739, w3685, w3724, w3739, w3682, w3738, w3739, w3679, w3742) -> (w3701:string)
                n2879 = Concatenate Strings(w3671, "," ("string"), w3659, w3661, w3660, w3743, w3746, w3660, w3744, w3745, w3671) -> (w3669:string)
                n2880 = local read "Tested by"() -> (w3675:string)
                n2881 = local read "String 33"() -> (w3676:string)
                n2882 = Concatenate Strings("," ("string"), "                                                                             " ("string")) -> (w3664:string)
                n2883 = Concatenate Strings(w3666, w3662, w3669, w3662, w3672, w3701, w3662, w3664, w3676, w3675) -> (→"export":string)
                n2884 = String To Path(string=w3703) -> (path=w3710:path)
                n2885 = local read "export"() -> (w3705:string)
                n2886 = call <vilib>:"Write Characters To File.vi"("append to file? (new file:F)"=FALSE, "character string"=w3705, "file path (dialog if empty)"=w3710) -> ()  [unwired: 2 in, 1 out]
              }
            }
          }
          frame Enabled {
          }
        }
        n2887 = case shown="True" "OK Button 17" {
          frame False {
          }
          frame True {
            (unwired) 0  # existing file
            w3963 = "Choose a datalog file to open"  # prompt
            n2888 = local write "OK Button 17"(FALSE ("OK Button 17")) -> ()
            n2889 = local read "String"() -> (w3958:string)
            n2890 = String To Path(string=w3958) -> (path=w3959:path)
            n2891 = File Dialog(6:"*.duf" ("pattern"), 7:w3963, 11:w3959) -> (0:w3950:errorcluster, 3:w3969:path)  [unwired: 4 in, 2 out]
            n2892 = Unbundle(w3950) -> ()  [unwired: 3 out]
            n2893 = Open/Create/Replace File "Open File"(file path (use dialog)=w3969) -> (refnum out=w3961:refnum<file>)  [unwired: 5 in, 2 out]
            n2894 = Strip Path(path=w3969) -> (name=w3967:string)  [unwired: 1 out]
            n2895 = Path To String(path=w3969) -> (string=w3952:string)
            n2896 = while {
              tunnel: w3961 -> [w3973]
              i -> [w3970]
              stop <- w3971 continue-if-true
              (unwired) TRUE ("line mode (F)")
              n2897 = Read from Text File "Read File"(file (use dialog)=w3973) -> (text=w3972:string)  [unwired: 3 in, 3 out]
